vi "DBedit-Queue-get.vi"(8 "error in (no error)":errorcluster, 11 "Gviewer in":refnum<class "DB-editor.lvclass">) -> (0 "error out":errorcluster, 1 "Time-out":bool, 2 "Query":T1, 3 "Gviewer out":refnum<class "DB-editor.lvclass">, 4 "# elements in queue":i32)   [LabVIEW 2020, in "Sgraph_lib_V1.lvlib" / "DB-editor.lvclass"]
doc: "Andre Koelewijn, 18 jan 2021\n\nReceive data from Queue"
uses:
  DB-editor.lvclass
  Gview/controls/Typedef_Gserver-Replies.ctl
  Gview/controls/Typedef_ServerActions.ctl
  DB-editor.lvclass/DB-editor.ctl
  Gview/Gviewer.lvclass
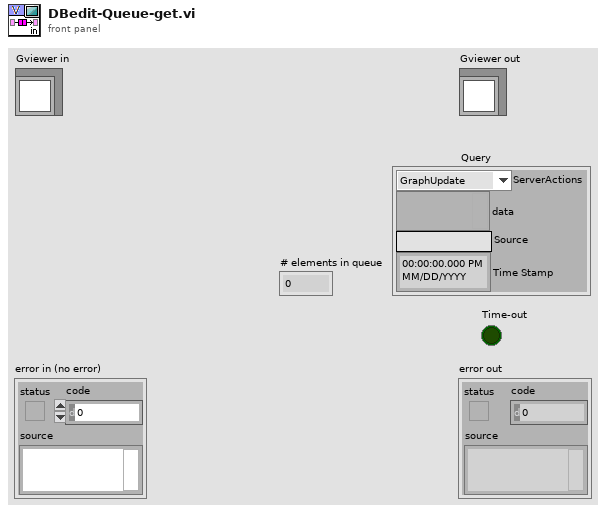
[diagram p1: front panel]
types:
  T1 = typedef "Typedef_Gserver-Replies.ctl" = cluster{"ServerActions":T2, "data":variant, "Source":string, "Time Stamp":timestamp}
  T2 = typedef "Sgraph_lib_V1.lvlib/Gviewer.lvclass/Typedef_ServerActions.ctl" = enum16{"GraphUpdate", "SendAllTags", "SendIniPath", "SetGeneralOptions", "EditTagsOpen", "EditTagsPresetSave", "EditTagsPresetLoad", "EditTagsClose", "NewTagSelection", "AutoScale", "DBeditStatus", "DBsaveConfirm", "GetXconstraints", "ExitGraph"}
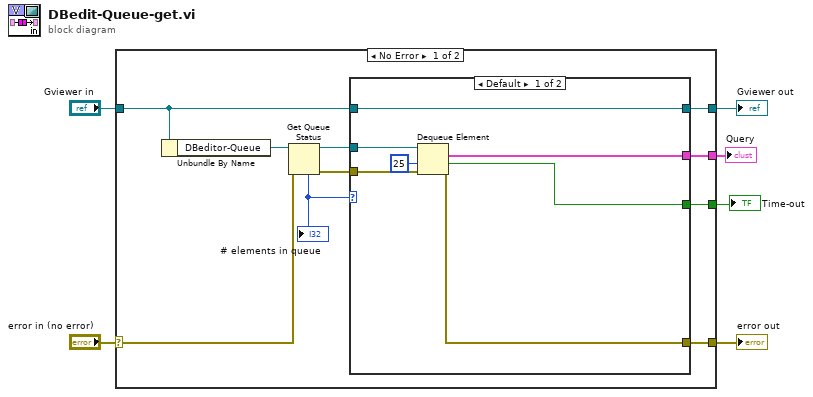
[diagram p0: block diagram]
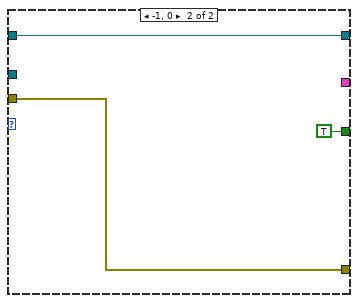
[diagram p2: hidden frame]
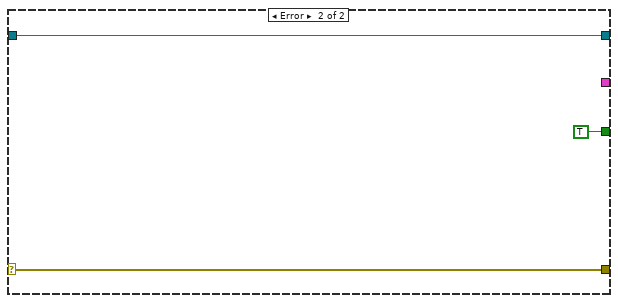
[diagram p3: hidden frame]
diagram:
  n1 = case shown="No Error" "error in (no error)" {
    selector: "error in (no error)" -> [w8 w29]
    tunnel: [w12 w29] -> w5
    tunnel: [w13 w28] -> w3
    tunnel: "Gviewer in" -> [w14 w28]
    tunnel: [w11 TRUE] -> w2
    tunnel: [w9 _] -> w1
    frame No Error {
      n2 = Unbundle By Name(w14) -> ("DBeditor-Queue"=w16:refnum<queue>)
      n3 = Get Queue Status(queue=w16, error in (no error)=w8) -> (queue out=w10:refnum<queue>, error out=w7:errorcluster, # elements in queue=w15:i32)  [unwired: 1 in, 5 out]
      "# elements in queue" <- w15
      n4 = case shown="Default" w15 {
        tunnel: w14 -> [w19 w26]
        tunnel: [w19 w26] -> w13
        tunnel: [w21 w24] -> w12
        tunnel: [w18 TRUE] -> w11
        tunnel: w10 -> [w22 _]
        tunnel: [w20 _] -> w9
        tunnel: w7 -> [w17 w24]
        frame Default {
          n5 = Dequeue Element(queue=w22, timeout in ms (-1)=25, error in (no error)=w17) -> (element=w20:T1, timed out?=w18:bool, error out=w21:errorcluster)  [unwired: 1 out]
        }
        frame -1, 0 {
        }
      }
    }
    frame Error {
    }
  }
  "error out" <- w5
  "Gviewer out" <- w3
  "Time-out" <- w2
  "Query" <- w1
